vi "WaveGraph Cursor.vi"(8 "エラー入力（エラーなし）":errorcluster, 9 "色":u32(colorbox), 10 "名称":string, 11 "WaveformGraph入力":refnum<vi>) -> (0 "エラー出力":errorcluster)   [LabVIEW 2014]
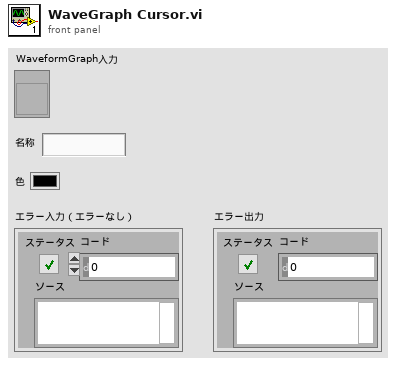
[diagram p1: front panel]
types:
  T1 = cluster{"Name":string, "Color":u32, "Style":u8, "Point Style":u8, "Name Visible":bool, "Allow Drag":bool, "Cursor Mode":u32, "Plot":i32, "Index":i32, "Position":cluster{"X":dbl, "Y":dbl}, "X Scale":u32, "Y Scale":u32, "Watch Plots":i32[], "Watch All Plots":bool, "Plot Area":i32, "Label Offset":cluster{"X":dbl, "Y":dbl}}
  T2 = typedef "LVCursorListTypeDef.ctl" = cluster{"Name":string, "Color":u32, "Style":u8, "Point Style":u8, "Name Visible":bool, "Allow Drag":bool, "Cursor Mode":u32, "Plot":i32, "Index":i32, "Position":cluster{"X":dbl, "Y":dbl}, "X Scale":u32, "Y Scale":u32, "Watch Plots":i32[], "Watch All Plots":bool, "Plot Area":i32, "Label Offset":cluster{"X":dbl, "Y":dbl}}[]
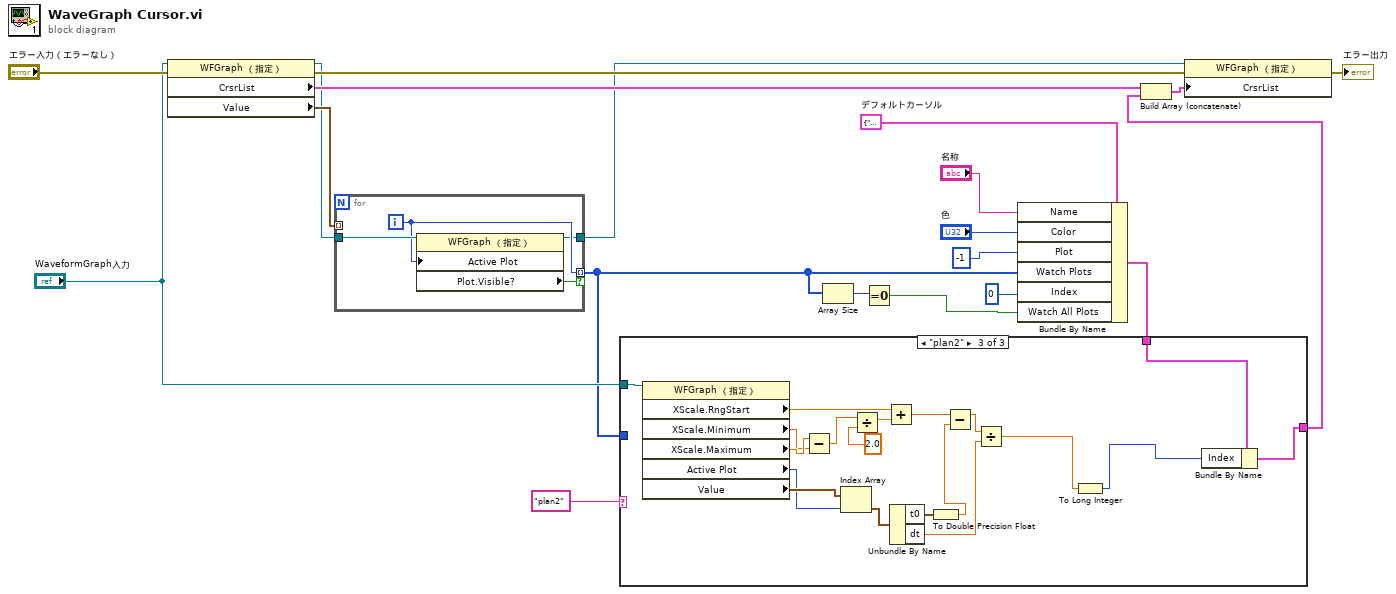
[diagram p0: block diagram]
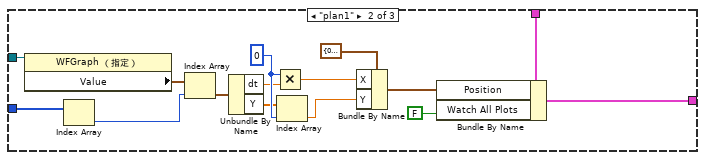
[diagram p3: hidden frame]
diagram:
  w11 = T1 {"Name"="カーソル0", "Color"=16776960, "Style"=2, "Point Style"=13, "Name Visible"=FALSE, "Allow Drag"=TRUE, "Cursor Mode"=2, "Plot"=-1, "Index"=42, "Position"={"X"=0.42, "Y"=43.0}, "X Scale"=0, "Y Scale"=0, "Watch Plots"=[], "Watch All Plots"=TRUE, "Plot Area"=0, "Label Offset"={"X"=-0.0012080536912751905, "Y"=172.10516252390056}}  # デフォルトカーソル
  n1 = property class="WFGraph （指定）"(reference="WaveformGraph入力", error in="エラー入力（エラーなし）") -> (reference out=w6:refnum<vi>, error out=w13:errorcluster, "CrsrList"=w19:T2, "Value"=w18:waveform(dbl)[])
  n2 = for {
    tunnel: w6 -> [w24]
    tunnel: w18 -> [_] mode=indexing
    tunnel: [w23] -> w3 mode=indexing if=w22
    tunnel: [w21] -> w7
    i -> [w23]
    n3 = property class="WFGraph （指定）"(reference=w24, "Active Plot"=w23) -> (reference out=w21:refnum<vi>, "Plot.Visible?"=w22:bool)  [unwired: 1 in, 1 out]
  }
  n4 = Array Size(array=w3) -> (size(s)=w2:i32)
  n5 = Equal To 0?(x=w2) -> (x = 0?=w1:bool)
  n6 = Bundle By Name(cluster=w11, "Name"="名称", "Color"="色", "Plot"=-1, "Watch Plots"=w3, "Index"=0, "Watch All Plots"=w1) -> (w9:T1)
  n7 = case shown="\"plan2\"" "plan2" {
    tunnel: w3 -> [_ w40 _]
    tunnel: w9 -> [w25 w28 w57]
    tunnel: [w25 w27 w56] -> w8
    tunnel: "WaveformGraph入力" -> [_ w26 w59]
    frame Default {
    }
    frame "plan1" {
      w38 = 0 ("Index")
      n8 = property class="WFGraph （指定）"(reference=w26) -> ("Value"=w32:waveform(dbl)[])  [unwired: 1 in, 2 out]
      n9 = Index Array(array=w40) -> (element=w33:i32)  [unwired: 1 in]
      n10 = Index Array(array=w32, index=w33) -> (element=w34:waveform(dbl))
      n11 = Unbundle By Name(w34) -> ("dt"=w37:dbl, "Y"=w35:dbl[])
      n12 = Multiply(x=w38, y=w37) -> (x*y=w39:dbl)
      n13 = Index Array(array=w35, index=w38) -> (element=w36:dbl)
      n14 = Bundle By Name(cluster=cluster{"X":dbl, "Y":dbl} {"X"=0.0, "Y"=0.0} ("Position"), "X"=w39, "Y"=w36) -> (w29:cluster{"X":dbl, "Y":dbl})
      n15 = Bundle By Name(cluster=w28, "Position"=w29, "Watch All Plots"=FALSE) -> (w27:T1)
    }
    frame "plan2" {
      n16 = property class="WFGraph （指定）"(reference=w59) -> ("XScale.RngStart"=w51:dbl, "XScale.Minimum"=w54:dbl, "XScale.Maximum"=w55:dbl, "Active Plot"=w49:u32, "Value"=w50:waveform(dbl)[])  [unwired: 1 in, 2 out]
      n17 = Subtract(x=w55, y=w54) -> (x-y=w53:dbl)
      n18 = Index Array(array=w50, index=w49) -> (element=w48:waveform(dbl))
      n19 = Divide(x=w53, y=2.0) -> (x/y=w52:dbl)
      n20 = Add(x=w51, y=w52) -> (x+y=w46:dbl)
      n21 = Unbundle By Name(w48) -> ("t0"=w44:timestamp, "dt"=w42:dbl)
      n22 = To Double Precision Float(number=w44) -> (double precision float=w43:dbl)
      n23 = Subtract(x=w46, y=w43) -> (x-y=w45:dbl)
      n24 = Divide(x=w45, y=w42) -> (x/y=w41:dbl)
      n25 = To Long Integer(number=w41) -> (32bit integer=w47:i32)
      n26 = Bundle By Name(cluster=w57, "Index"=w47) -> (w56:T1)
    }
  }
  n27 = Build Array (concatenate)(w19, w8) -> (w15:T2)
  n28 = property class="WFGraph （指定）"(reference=w7, error in=w13, "CrsrList"=w15) -> (error out=→"エラー出力":errorcluster)  [unwired: 1 out]
